vi "SOAE-Get Next Data File.vi"(0 "Expt State":T1) -> (4 "Run #":i32, 8 "Path":path)   [LabVIEW 2020]
uses:
  CFTS Main Panel SubVIs/CFTS-Experiment State.ctl
  <vilib>/regexp/Match Regular Expression.xnode
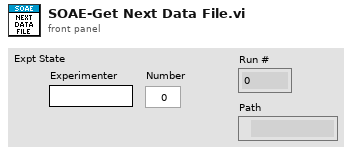
[diagram p1: front panel]
types:
  T1 = typedef "CFTS-Experiment State.ctl" = cluster{"Experimenter":string, "Number":u32, "Right":string, "Left":string, "Data Folder":path, "State File":path, "Version Info":string, "End Exposure Time":dbl, "Exposure Duration":string, "Run #":cluster{"CAP":i16, "ABR":i16, "DP":i16, "VsEP":i16, "MeasSeq":i16, "SubSeq":i16, "SFOAE":i16}}
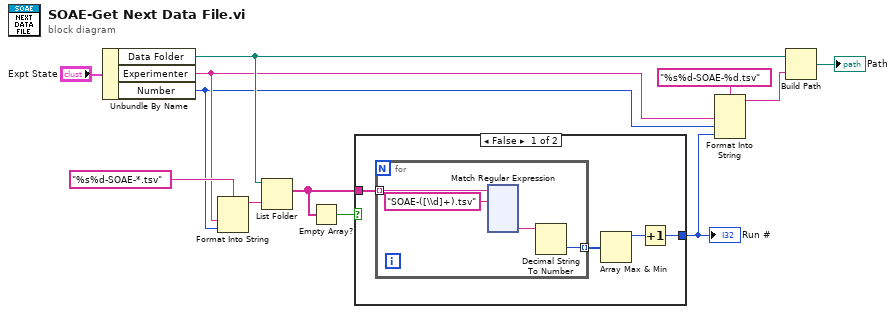
[diagram p0: block diagram]
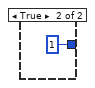
[diagram p2: hidden frame]
diagram:
  n1 = Unbundle By Name("Expt State") -> ("Data Folder"=w7:path, "Experimenter"=w5:string, "Number"=w4:u32)
  n2 = Format Into String(format string="%s%d-SOAE-*.tsv", w5, w4) -> (resulting string=w10:string)  [unwired: 2 in, 1 out]
  n3 = List Folder(path=w7, pattern=w10) -> (filenames=w9:string[])  [unwired: 2 in, 3 out]
  n4 = Empty Array?(array=w9) -> (empty?=w8:bool)
  n5 = case shown="False" w8 {
    tunnel: w9 -> [w16 _]
    tunnel: [w13 1] -> w1
    frame False {
      n6 = for {
        tunnel: w16 -> [w20] mode=indexing
        tunnel: [w17] -> w15 mode=indexing
        n7 = xnode "Match Regular Expression"("input string"=w20, "regular expression"="SOAE-([\\d]+).tsv") -> ("submatch 1"=w18:string)  [unwired: 4 in, 5 out]
        n8 = Decimal String To Number(string=w18) -> (number=w17:i32)  [unwired: 2 in, 1 out]
      }
      n9 = Array Max & Min(array=w15) -> (max value=w14:i32)  [unwired: 3 out]
      n10 = Increment(x=w14) -> (x+1=w13:i32)
    }
    frame True {
    }
  }
  "Run #" <- w1
  n11 = Format Into String(format string="%s%d-SOAE-%d.tsv", w5, w4, w1) -> (resulting string=w3:string)  [unwired: 2 in, 1 out]
  n12 = Build Path(base path=w7, name or relative path=w3) -> (appended path=→"Path":path)
